vi "Get Relay numbers 340-LEPL-102-A.vi"(8 "error in (no error)":errorcluster) -> (0 "error out":errorcluster, 2 "DUT2":T1, 3 "DUT1":T1)   [LabVIEW 2023]
uses:
  DUT_Relays_340-LEPL-102-A.ctl
  <vilib>/Utility/config.llb/Read Key (U32).vi
  <vilib>/Utility/config.llb/NI_LVConfig.lvlib
panel:
  out "error IO":errorcluster
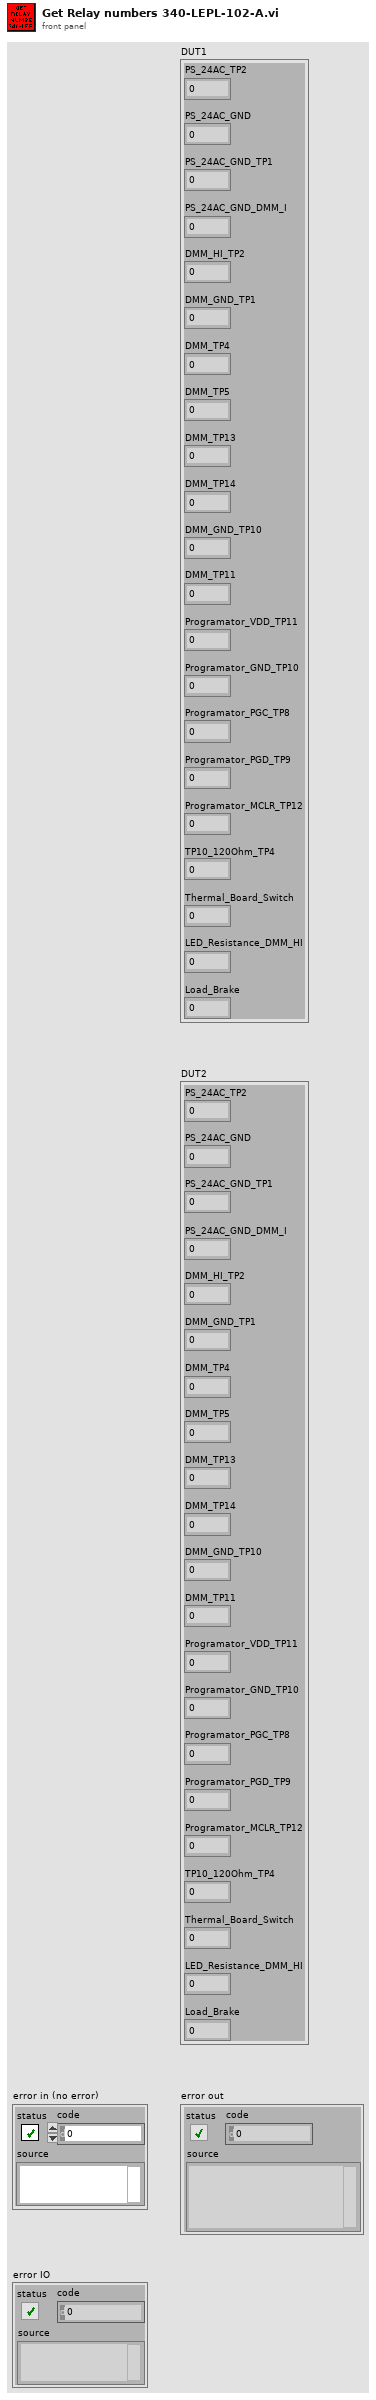
[diagram p1: front panel]
types:
  T1 = typedef "DUT_Relays_340-LEPL-102-A.ctl" = cluster{"PS_24AC_TP2":i32, "PS_24AC_GND":i32, "PS_24AC_GND_TP1":i32, "PS_24AC_GND_DMM_I":i32, "DMM_HI_TP2":i32, "DMM_GND_TP1":i32, "DMM_TP4":i32, "DMM_TP5":i32, "DMM_TP13":i32, "DMM_TP14":i32, "DMM_GND_TP10":i32, "DMM_TP11":i32, "Programator_VDD_TP11":i32, "Programator_GND_TP10":i32, "Programator_PGC_TP8":i32, "Programator_PGD_TP9":i32, "Programator_MCLR_TP12":i32, "TP10_120Ohm_TP4":i32, "Thermal_Board_Switch":i32, "LED_Resistance_DMM_HI":i32, "Load_Brake":i32}
  T2 = typedef "NI_LVConfig.lvlib/Config Data RefNum.ctl" = refnum<k1>
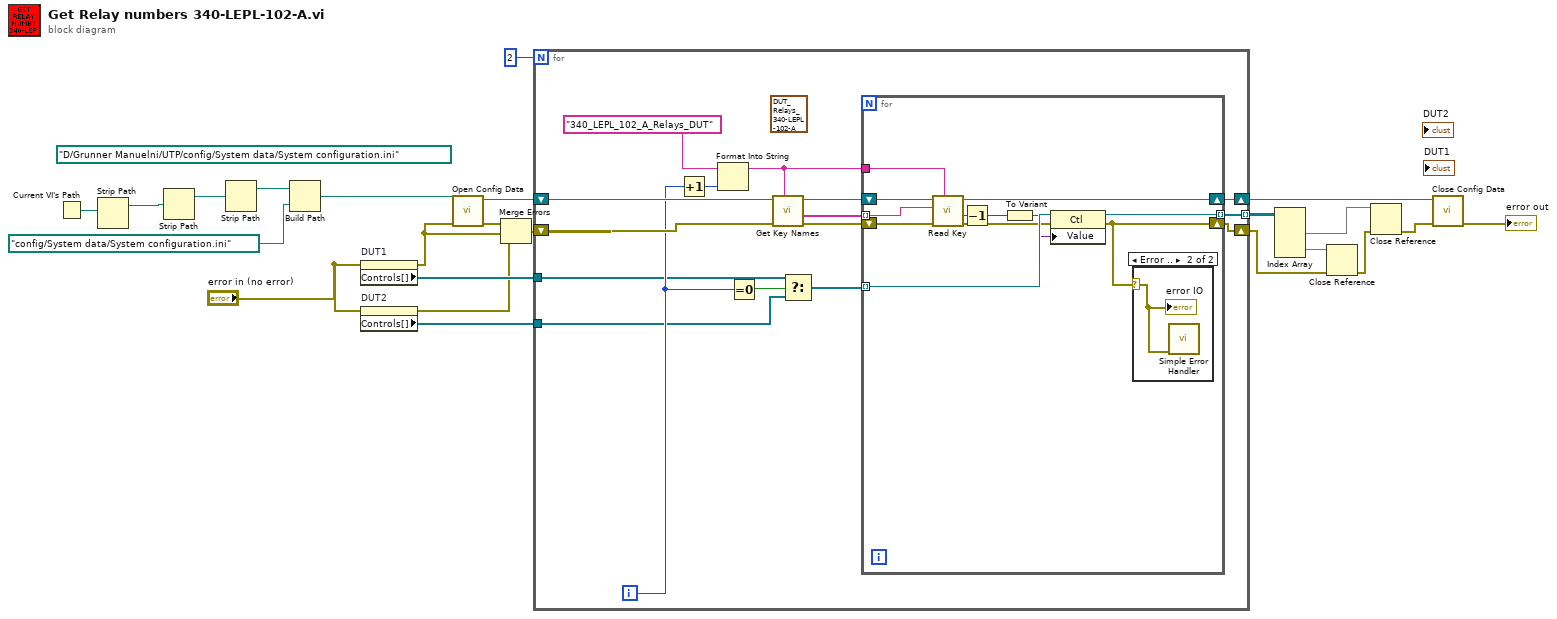
[diagram p0: block diagram]
diagram:
  (unwired) path "D:/Grunner Manuelni/UTP/config/System data/System configuration.ini" ("configuration file path")
  n1 = Current VI's Path() -> (path=w4:path)
  n2 = Strip Path(path=w4) -> (stripped path=w3:path)  [unwired: 1 out]
  n3 = Strip Path(path=w3) -> (stripped path=w7:path)  [unwired: 1 out]
  n4 = Strip Path(path=w7) -> (stripped path=w6:path)  [unwired: 1 out]
  n5 = Build Path(base path=w6, name or relative path=path "config/System data/System configuration.ini") -> (appended path=w2:path)
  n6 = property on="DUT1" class="Clust (strict)"(error in="error in (no error)") -> (error out=w1:errorcluster, "Controls[]"=w18:refnum<vi>[])  [unwired: 1 in, 1 out]
  n7 = property on="DUT2" class="Clust (strict)"(error in="error in (no error)") -> (error out=w14:errorcluster, "Controls[]"=w17:refnum<vi>[])  [unwired: 1 in, 1 out]
  n8 = call <vilib>:"Open Config Data.vi"("error in (no error)"=w1, "configuration file path"=w2) -> ("error out"=w15:errorcluster, "refnum"=w23:T2)  [unwired: 7 in, 1 out]
  n9 = Merge Errors(w15, w1, w14) -> (w16:errorcluster)
  n10 = for {
    N: 2 -> [_]
    shift-right: [w33] -> w22
    shift-left: w23 -> [w39]
    shift-right: [w34] -> w8
    shift-left: w16 -> [w36]
    tunnel: w18 -> [w28]
    tunnel: w17 -> [w25]
    tunnel: [w24] -> w12 mode=indexing
    i -> [w29]
    (unwired) T1 {"PS_24AC_TP2"=0, "PS_24AC_GND"=0, "PS_24AC_GND_TP1"=0, "PS_24AC_GND_DMM_I"=0, "DMM_HI_TP2"=0, "DMM_GND_TP1"=0, "DMM_TP4"=0, "DMM_TP5"=0, "DMM_TP13"=0, "DMM_TP14"=0, "DMM_GND_TP10"=0, "DMM_TP11"=0, "Programator_VDD_TP11"=0, "Programator_GND_TP10"=0, "Programator_PGC_TP8"=0, "Programator_PGD_TP9"=0, "Programator_MCLR_TP12"=0, "TP10_120Ohm_TP4"=0, "Thermal_Board_Switch"=0, "LED_Resistance_DMM_HI"=0, "Load_Brake"=0} ("DUT1")
    n11 = Increment(x=w29) -> (x+1=w31:i32)
    n12 = Format Into String(initial string="340_LEPL_102_A_Relays_DUT" ("section"), w31) -> (resulting string=w30:string)  [unwired: 2 in, 1 out]
    n13 = Equal To 0?(x=w29) -> (x = 0?=w26:bool)
    n14 = call <vilib>:"Get Key Names.vi"("section"=w30, "error in (no error)"=w36, "refnum"=w39) -> ("error out"=w35:errorcluster, "key names"=w38:string[], "refnum out"=w37:T2)  [unwired: 5 in, 1 out]
    n15 = Select(t=w28, s=w26, f=w25) -> (s? t:f=w27:refnum<vi>[])
    n16 = for {
      tunnel: w38 -> [w49] mode=indexing
      shift-right: [w50] -> w33
      shift-left: w37 -> [w51]
      tunnel: w30 -> [w48]
      tunnel: w27 -> [w46] mode=indexing
      tunnel: [w42] -> w24 mode=indexing
      shift-right: [w41] -> w34
      shift-left: w35 -> [w47]
      n17 = call-poly <vilib>:"Read Key.vi"("section"=w48, "error in (no error)"=w47, "key"=w49, "refnum"=w51) -> ("error out"=w45:errorcluster, "value"=w44:u32, "refnum out"=w50:T2)  [unwired: 4 in, 1 out]
      n18 = Decrement(x=w44) -> (x-1=w40:u32)
      n19 = To Variant(anything=w40) -> (Variant=w43:variant)
      n20 = property class="Ctl"(reference=w46, error in=w45, "Value"=w43) -> (reference out=w42:refnum<vi>, error out=w41:errorcluster)
      n21 = case shown="Error .." w41 {
        selector: w41 -> [_ w52]
        frame No Error {
        }
        frame Error {
          n22 = call <vilib>:"Simple Error Handler.vi"("error in (no error)"=w52) -> ()  [unwired: 4 in, 5 out]
          "error IO" <- w52
        }
      }
    }
  }
  n23 = Index Array(array=w12) -> (element #1=w11:refnum<vi>[], element #2=w10:refnum<vi>[])  [unwired: 4 in]
  n24 = Close Reference(reference=w10, error in (no error)=w8) -> (error out=w9:errorcluster)
  n25 = Close Reference(reference=w11, error in (no error)=w9) -> (error out=w21:errorcluster)
  n26 = call <vilib>:"Close Config Data.vi"("error in (no error)"=w21, "refnum"=w22) -> ("error out"=→"error out":errorcluster)  [unwired: 8 in, 1 out]
